vi "Search Sensor.vi"(8 "error in (no error)":errorcluster, 9 "pNumberofSensor":u32, 10 "pSensorIP":u32, 11 "nHostIP":u32) -> (0 "error out":errorcluster, 1 "pNumberofSensor out":u32, 2 "pSensorIP out":u32, 3 "function return":i32)   [LabVIEW 2017, in "imgAcquisition.lvlib"]
doc: "DLLFunction int __stdcall ImageCapSearchSensor(unsigned int nHostIP, unsigned int* pSensorIP, unsigned int* pNumberofSensor);"
uses:
  imgAcquisition.lvlib
  lib/ImageCaptureDLL.dll
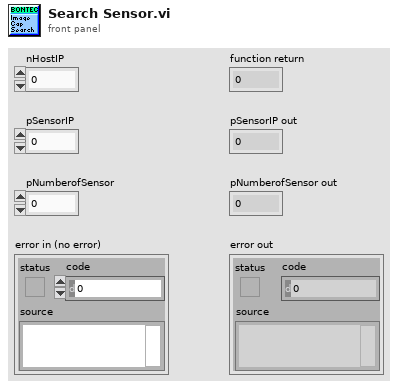
[diagram p1: front panel]
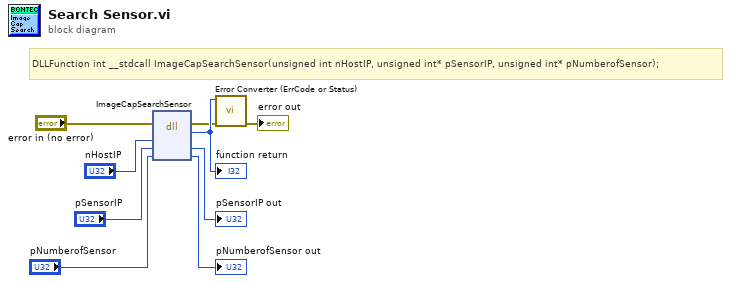
[diagram p0: block diagram]
diagram:
  # "DLLFunction int __stdcall ImageCapSearchSensor(unsigned int nHostIP, unsigned int* pSensorIP, unsigned int* pNumberofSensor);"
  n1 = dll-call lib="F:/BonTechFlatPanelLVDriver/lib/ImageCaptureDLL.*" fn="ImageCapSearchSensor"(error in="error in (no error)", "nHostIP"="nHostIP", "pSensorIP"="pSensorIP", "pNumberofSensor"="pNumberofSensor") -> (error out=w2:errorcluster, w9:i32, "pSensorIP"=→"pSensorIP out":u32, "pNumberofSensor"=→"pNumberofSensor out":u32)  [unwired: 3 in, 1 out]
  "function return" <- w9
  n2 = call "Error Converter (ErrCode or Status).vi"("error in (no error)"=w2, "error code"=w9) -> ("error out"=→"error out":errorcluster)  [unwired: 9 in]
